vi "Handle Error.vi"(8 "error in (no error)":errorcluster, 11 "Error Reporter in":refnum<class "Error Reporter.lvclass">) -> (0 "error out":errorcluster, 2 "stop actor?":bool=TRUE, 3 "Error Reporter out":refnum<class "Error Reporter.lvclass">)   [LabVIEW 2024, in "Error Reporter.lvlib" / "Error Reporter.lvclass"]
doc: "<p>(<strong>Filename</strong>: <span class=\"dnl\">Actor Framework.lvlib:Actor.lvclass:Handle Error.vi</span>)</p>\n<p>Defines how the actor handles an error that occurred while processing a message. By default, this method does nothing except stop the actor.</p>"
uses:
  Error Reporter.lvclass
  Error Reporter.lvclass/Error Reporter.ctl
  ~Error/~Error Messages/Error Msg/Error Msg.lvclass/Error Msg.ctl
  <vilib>/ActorFramework/Message Enqueuer/Message Enqueuer.lvclass/Message Enqueuer.ctl
  <vilib>/ActorFramework/Message Enqueuer/Enqueue.vi
  ~Error/~Error Messages/Error Msg/Error Msg.lvclass
  C:/Program Files (x86)/National Instruments/LabVIEW 2024/vi.lib/ActorFramework/Message/Message.lvclass
  <vilib>/ActorFramework/Message Priority Queue/Priority Enqueue.vi
  <vilib>/ActorFramework/Actor/Actor.lvclass
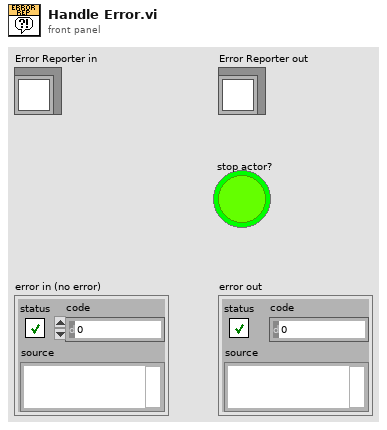
[diagram p1: front panel]
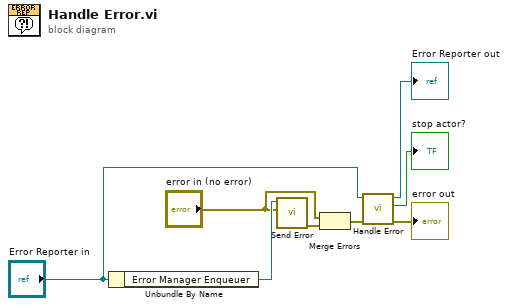
[diagram p0: block diagram]
diagram:
  n1 = Unbundle By Name("Error Reporter in") -> ("Error Manager Enqueuer"=w6:refnum<class "Message Enqueuer.lvclass">)
  n2 = call "Send Error.vi"("error"="error in (no error)", "Message Enqueuer"=w6) -> ("error out"=w2:errorcluster)  [unwired: 8 in, 1 out]
  n3 = Merge Errors("error in (no error)", w2) -> (w1:errorcluster)
  n4 = call-parent "Handle Error.vi"("error in (no error)"=w1, "Actor in"="Error Reporter in") -> ("error out"=→"error out":errorcluster, "stop actor?"=→"stop actor?":bool, "Actor out"=→"Error Reporter out":refnum<class "Error Reporter.lvclass">)  [unwired: 7 in]
